vi "Set Security Level CORE.vi"(8 "error in (no error)":errorcluster, 9 "Set or Clear":T1, 10 "Security Level":T2, 11 "Motion Detectors in":refnum<class "Motion Detectors.lvclass">) -> (0 "error out":errorcluster, 2 "Last Action Performed":string, 3 "Motion Detectors out":refnum<class "Motion Detectors.lvclass">)   [LabVIEW 2020, in "Motion Detectors.lvclass"]
uses:
  Motion Detectors.lvclass
  Security System/Security Level.ctl
  Security System/Set or Clear.ctl
  Motion Detectors.lvclass/Motion Detectors.ctl
  Mode.ctl
  Security System/Security System.lvclass
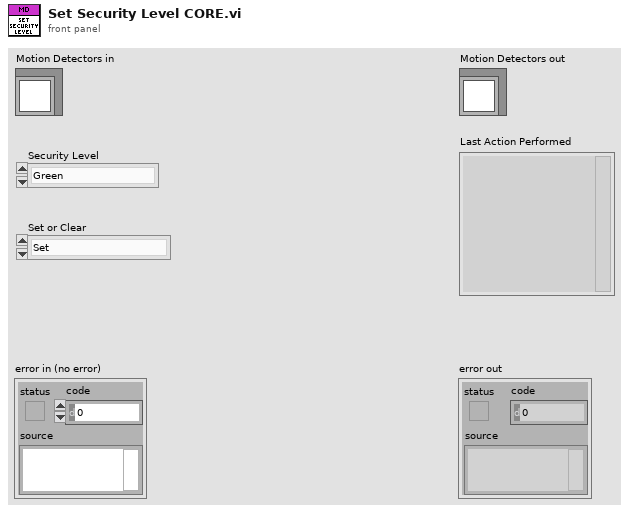
[diagram p1: front panel]
types:
  T1 = typedef "Security System.lvclass/Set or Clear.ctl" = enum16{"Set", "Clear"}
  T2 = typedef "Security System.lvclass/Security Level.ctl" = enum16{"Green", "Yellow", "Orange", "Red"}
  T3 = typedef "Motion Detectors.lvclass/Mode.ctl" = enum16{"Visual Spectrum", "Infrared +  Visual", "Infrared + Heat +Visual"}
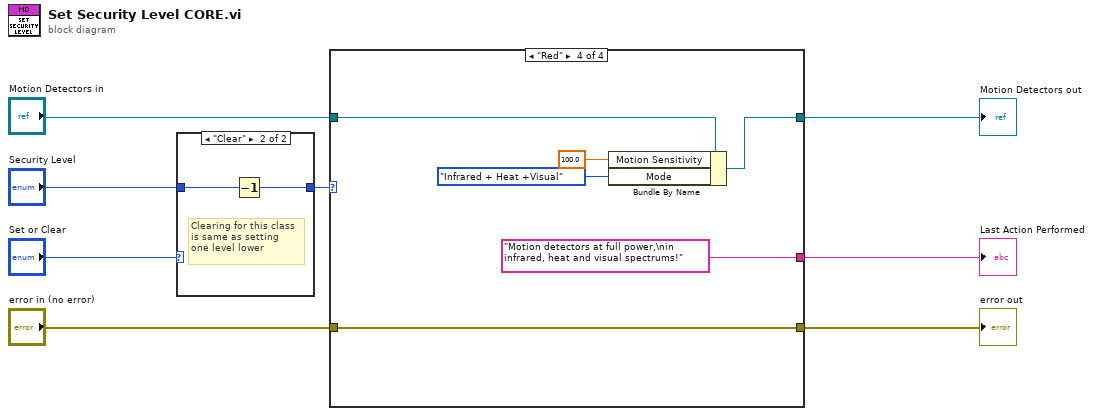
[diagram p0: block diagram]
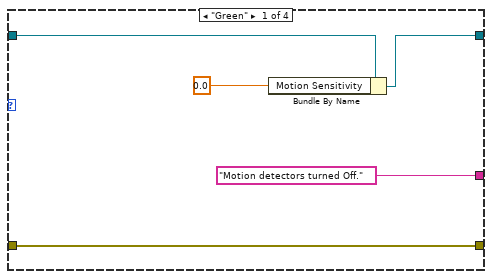
[diagram p2: hidden frame]
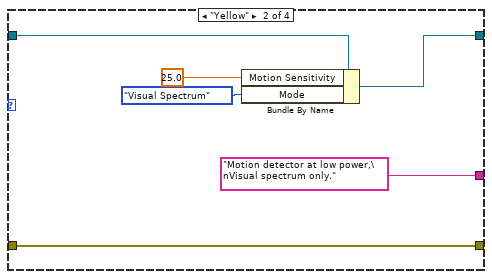
[diagram p3: hidden frame]
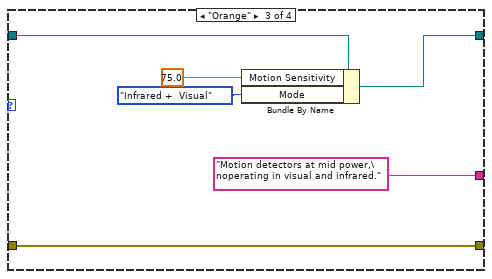
[diagram p4: hidden frame]
diagram:
  n1 = case shown="\"Clear\"" "Set or Clear" {
    tunnel: "Security Level" -> [w9 w11]
    tunnel: [w9 w10] -> w8
    frame "Set" {
    }
    frame "Clear" {
      # "Clearing for this class\nis same as setting\none level lower"
      n2 = Decrement(x=w11) -> (x-1=w10:T2)
    }
  }
  n3 = case shown="\"Red\"" w8 {
    tunnel: "Motion Detectors in" -> [w16 w22 w28 w34]
    tunnel: "error in (no error)" -> [w12 w19 w25 w32]
    tunnel: [w15 w21 w27 w33] -> w5
    tunnel: ["Motion detectors turned Off." "Motion detector at low power,\nVisual spectrum only." "Motion detectors at mid power,\noperating in visual and infrared." "Motion detectors at full power,\nin infrared, heat and visual spectrums!"] -> w4
    tunnel: [w12 w19 w25 w32] -> w3
    frame "Green" {
      n4 = Bundle By Name(cluster=w16, "Motion Sensitivity"=0.0 ("Metal Detector Sensitivity")) -> (w15:refnum<class "Motion Detectors.lvclass">)
    }
    frame "Yellow" {
      n5 = Bundle By Name(cluster=w22, "Motion Sensitivity"=25.0 ("Metal Detector Sensitivity"), "Mode"=Mode."Visual Spectrum") -> (w21:refnum<class "Motion Detectors.lvclass">)
    }
    frame "Orange" {
      n6 = Bundle By Name(cluster=w28, "Motion Sensitivity"=75.0 ("Metal Detector Sensitivity"), "Mode"=Mode."Infrared +  Visual") -> (w27:refnum<class "Motion Detectors.lvclass">)
    }
    frame "Red" {
      n7 = Bundle By Name(cluster=w34, "Motion Sensitivity"=100.0, "Mode"=Mode."Infrared + Heat +Visual") -> (w33:refnum<class "Motion Detectors.lvclass">)
    }
  }
  "error out" <- w3
  "Motion Detectors out" <- w5
  "Last Action Performed" <- w4
